vi "swerve_open_module.vi"(0 "Module Suffix":string, 5 "Drive CAN ID":u8, 7 "Azimuth CAN ID":u8, 9 "Encoder CAN ID":u8, 11 "error in":errorcluster, 12 "Encoder Offset (Deg)":dbl) -> (15 "error out":errorcluster)   [LabVIEW 2020]
uses:
  <vilib>/Rock Robotics/WPI/ThirdParty/Phoenix-LabVIEW/CANCoder/Controls/CTRE_Phoenix_CANcoder_SensorInitializationStrategy.ctl
  <vilib>/Rock Robotics/WPI/ThirdParty/Phoenix-LabVIEW/Motor Controller/Controls/CTRE_Phoenix_MotorControl_NeutralMode.ctl
  <vilib>/Rock Robotics/WPI/ThirdParty/Phoenix-LabVIEW/Motor Controller/Controls/CTRE_Phoenix_MotorControl_RemoteSourceType.ctl
  <vilib>/Rock Robotics/WPI/ThirdParty/Phoenix-LabVIEW/Motor Controller/Controls/CTRE_Phoenix_MotorControl_FeedbackDevice_TalonFX.ctl
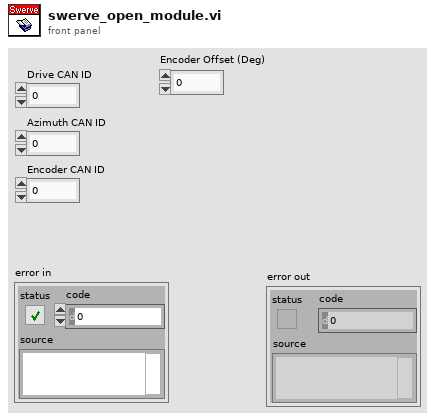
[diagram p1: front panel]
types:
  T1 = typedef "CTRE_Phoenix_MotorControl_NeutralMode.ctl" = enum8{"EEPROMSetting", "Override to Coast", "Override to Brake"}
  T2 = typedef "CTRE_Phoenix_MotorControl_FeedbackDevice_TalonFX.ctl" = i8
  T3 = typedef "CTRE_Phoenix_MotorControl_RemoteSourceType.ctl" = enum16{"Off", "Talon SRX Selected Sensor", "Pigeon IMU Yaw", "Pigeon IMU Pitch", "Pigeon IMU Roll", "CANifier Quadrature", "CANifier PWM Input 0", "CANifier PWM Input 1", "CANifier PWM Input 2", "CANifier PWM Input 3", "Gadgeteer Pigeon Yaw", "Gadgeteer Pigeon Pitch", "Gadgeteer Pigeon Roll", "CANCoder"}
  T4 = typedef "CTRE_Phoenix_CANcoder_SensorInitializationStrategy.ctl" = enum16{"Boot To Zero", "Boot To Absolute Position"}
  T5 = typedef "WPI_MotorControlDeviceRef.ctl" = cluster{"DeviceStatus":errorcluster, "Type":T6, "PWM":cluster{"PWM Channel":T7, "DeadBand":T8}, "CAN":cluster{"Device Number":u8, "SetOutput VI Ref":variant, "GetOutput VI Ref":variant, "Enable VI Ref":variant, "Disable VI Ref":variant, "Data":variant}, "Invert":bool, "DIO PWM":cluster{"PWM \"Enable\" Channel":T7, "DIOChannel":T9, "PWM Rate":dbl}}
  T6 = typedef "WPI_MotorControlType.ctl" = enum16{"PWM", "CAN", "DIO PWM"}
  T7 = typedef "FPGA_DIOPWMChannel.ctl" = enum8{"PWM 0", "PWM 1", "PWM 2", "PWM 3", "PWM 4", "PWM 5", "PWM 6", "PWM 7", "PWM 8", "PWM 9", "PWM MXP 0", "PWM MXP 1", "PWM MXP 2", "PWM MXP 3", "PWM MXP 4", "PWM MXP 5", "PWM MXP 6", "PWM MXP 7", "PWM MXP 8", "PWM MXP 9", "Invalid"}
  T8 = typedef "WPI_PWMDeadband.ctl" = cluster{"Name":string, "maxPositivePwm":i32, "minPositivePwm":i32, "centerPwm":i32, "maxNegativePwm":i32, "minNegativePwm":i32, "angularRange":u16}
  T9 = typedef "FPGA_DIOChannel.ctl" = enum8{"DIO 0", "DIO 1", "DIO 2", "DIO 3", "DIO 4", "DIO 5", "DIO 6", "DIO 7", "DIO 8", "DIO 9", "DIO MXP 0", "DIO MXP 1", "DIO MXP 2", "DIO MXP 3", "DIO MXP 4", "DIO MXP 5", "DIO MXP 6", "DIO MXP 7", "DIO MXP 8", "DIO MXP 9", "DIO MXP 10", "DIO MXP 11", "DIO MXP 12", "DIO MXP 13", "DIO MXP 14", "DIO MXP 15", "SPI Port CS1", "SPI Port CS2", "SPI Port CS3", "SPI Port MISO", "SPI Port MOSI", "Invalid"}
  T10 = typedef "CTRE_Phoenix_CANcoder_DeviceRef.ctl" = cluster{"DeviceStatus":errorcluster, "Device Number":u8, "Handle":u64, "UsageFrame":u32, "Library Path":path}
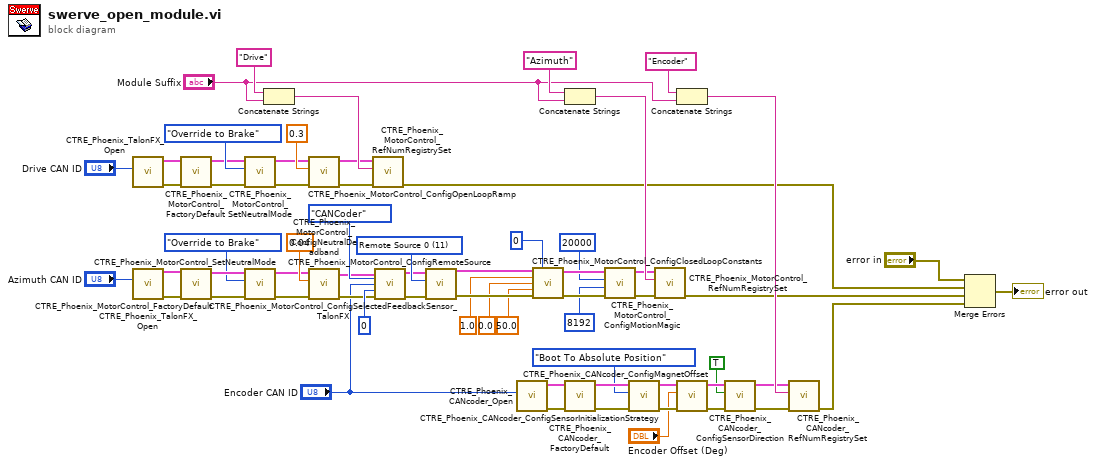
[diagram p0: block diagram]
diagram:
  w42 = T2 11 items=["Integrated Sensor"=1, "Sensor Sum (S0 + S1)"=9, "Sensor Difference (D0 - D1)"=10, "Remote Source 0"=11, "Remote Source 1"=12, "None"=14, "Software Emulated"=15] ("Talon FX Feedback Device")
  n1 = call <vilib>:"CTRE_Phoenix_TalonFX_Open.vi"("Device Number"="Drive CAN ID") -> ("error out"=w60:errorcluster, "PhoenixMotorControlDevRef"=w61:T5)  [unwired: 9 in]
  n2 = call <vilib>:"CTRE_Phoenix_TalonFX_Open.vi"("Device Number"="Azimuth CAN ID") -> ("error out"=w59:errorcluster, "PhoenixMotorControlDevRef"=w58:T5)  [unwired: 9 in]
  n3 = call <vilib>:"CTRE_Phoenix_MotorControl_FactoryDefault.vi"("error in"=w60, "PhoenixMotorControlDevRef"=w61) -> ("error out"=w11:errorcluster, "PhoenixMotorControlDevRef"=w12:T5)  [unwired: 8 in]
  n4 = call <vilib>:"CTRE_Phoenix_MotorControl_FactoryDefault.vi"("error in"=w59, "PhoenixMotorControlDevRef"=w58) -> ("error out"=w30:errorcluster, "PhoenixMotorControlDevRef"=w31:T5)  [unwired: 8 in]
  n5 = call <vilib>:"CTRE_Phoenix_MotorControl_SetNeutralMode.vi"("error in (no error)"=w11, "Motor Control Neutral Mode"=CTRE_Phoenix_MotorControl_NeutralMode."Override to Brake", "PhoenixMotorControlDevRef"=w12) -> ("error out"=w9:errorcluster, "PhoenixMotorControlDevRef"=w10:T5)  [unwired: 7 in]
  n6 = call <vilib>:"CTRE_Phoenix_MotorControl_SetNeutralMode.vi"("error in (no error)"=w30, "Motor Control Neutral Mode"=CTRE_Phoenix_MotorControl_NeutralMode."Override to Brake", "PhoenixMotorControlDevRef"=w31) -> ("error out"=w28:errorcluster, "PhoenixMotorControlDevRef"=w29:T5)  [unwired: 7 in]
  n7 = Concatenate Strings("Drive" ("string"), "Module Suffix") -> (w62:string)
  n8 = call <vilib>:"CTRE_Phoenix_MotorControl_ConfigOpenLoopRamp.vi"("error in (no error)"=w9, "secondsFromNeutralToFull"=0.3 ("Drive Ramp (Sec)"), "PhoenixMotorControlDevRef"=w10) -> ("error out"=w7:errorcluster, "PhoenixMotorControlDevRef"=w8:T5)  [unwired: 7 in]
  n9 = call <vilib>:"CTRE_Phoenix_MotorControl_ConfigNeutralDeadband.vi"("error in (no error)"=w28, "Percent Deadband"=0.04, "PhoenixMotorControlDevRef"=w29) -> ("error out"=w25:errorcluster, "PhoenixMotorControlDevRef"=w26:T5)  [unwired: 7 in]
  n10 = call <vilib>:"CTRE_Phoenix_MotorControl_RefNumRegistrySet.vi"("error in (no error)"=w7, "refnum name"=w62, "PhoenixMotorControlDevRef"=w8) -> ("error out"=w5:errorcluster)  [unwired: 7 in, 1 out]
  n11 = call <vilib>:"CTRE_Phoenix_MotorControl_ConfigRemoteSource.vi"("PhoenixMotorControlDevRef"=w26, "Remote Device Type"=CTRE_Phoenix_MotorControl_RemoteSourceType."CANCoder", "Remote Device ID"="Encoder CAN ID", "Source Index (0/1)"=u32 0, "error in (no error)"=w25) -> ("PhoenixMotorControlDevRef"=w39:T5, "error out"=w38:errorcluster)  [unwired: 9 in]
  n12 = call <vilib>:"CTRE_Phoenix_MotorControl_ConfigSelectedFeedbackSensor_TalonFX.vi"("error in (no error)"=w38, "Talon FX Feedback Device"=w42, "PhoenixMotorControlDevRef"=w39) -> ("error out"=w23:errorcluster, "PhoenixMotorControlDevRef"=w24:T5)  [unwired: 7 in]
  n13 = call <vilib>:"CTRE_Phoenix_CANcoder_Open.vi"("Device Number"="Encoder CAN ID") -> ("error out"=w35:errorcluster, "CTRE_CANcoder_DeviceRef"=w36:T10)  [unwired: 9 in]
  n14 = call <vilib>:"CTRE_Phoenix_MotorControl_ConfigClosedLoopConstants.vi"("PhoenixMotorControlDevRef"=w24, "slotIdx"=0, "P"=1.0, "I"=0.0 ("P"), "D"=50.0 ("P"), "error in (no error)"=w23) -> ("PhoenixMotorControlDevRef"=w18:T5, "error out"=w17:errorcluster)  [unwired: 8 in]
  n15 = Concatenate Strings("Azimuth" ("string"), "Module Suffix") -> (w55:string)
  n16 = call <vilib>:"CTRE_Phoenix_CANcoder_FactoryDefault.vi"("error in"=w35, "CTRE_CANcoder_DeviceRef"=w36) -> ("error out"=w52:errorcluster, "CTRE_CANcoder_DeviceRef"=w51:T10)  [unwired: 8 in]
  n17 = call <vilib>:"CTRE_Phoenix_MotorControl_ConfigMotionMagic.vi"("error in (no error)"=w17, "Acceleration"=8192 ("Cruise Velocity"), "Cruise Velocity"=20000, "PhoenixMotorControlDevRef"=w18) -> ("error out"=w13:errorcluster, "PhoenixMotorControlDevRef"=w14:T5)  [unwired: 6 in]
  n18 = call <vilib>:"CTRE_Phoenix_CANcoder_ConfigSensorInitializationStrategy.vi"("error in"=w52, "Sensor Initialization Strategy"=CTRE_Phoenix_CANcoder_SensorInitializationStrategy."Boot To Absolute Position", "CTRE_CANcoder_DeviceRef"=w51) -> ("error out"=w48:errorcluster, "CTRE_CANcoder_DeviceRef"=w47:T10)  [unwired: 7 in]
  n19 = call <vilib>:"CTRE_Phoenix_MotorControl_RefNumRegistrySet.vi"("error in (no error)"=w13, "refnum name"=w55, "PhoenixMotorControlDevRef"=w14) -> ("error out"=w4:errorcluster)  [unwired: 7 in, 1 out]
  n20 = Concatenate Strings("Encoder" ("string"), "Module Suffix") -> (w53:string)
  n21 = call <vilib>:"CTRE_Phoenix_CANcoder_ConfigMagnetOffset.vi"("error in"=w48, "Magnet Offset (Degrees)"="Encoder Offset (Deg)", "CTRE_CANcoder_DeviceRef"=w47) -> ("error out"=w45:errorcluster, "CTRE_CANcoder_DeviceRef"=w44:T10)  [unwired: 7 in]
  n22 = call <vilib>:"CTRE_Phoenix_CANcoder_ConfigSensorDirection.vi"("error in"=w45, "Sensor Direction"=TRUE, "CTRE_CANcoder_DeviceRef"=w44) -> ("error out"=w33:errorcluster, "CTRE_CANcoder_DeviceRef"=w34:T10)  [unwired: 7 in]
  n23 = call <vilib>:"CTRE_Phoenix_CANcoder_RefNumRegistrySet.vi"("error in (no error)"=w33, "refnum name"=w53, "CTRE_CANcoder_DeviceRef"=w34) -> ("error out"=w3:errorcluster)  [unwired: 7 in, 1 out]
  n24 = Merge Errors("error in", w5, w4, w3) -> (→"error out":errorcluster)
